vi "get User Info List.vi"(8 "error in (no error)":errorcluster, 11 "[Data] Abstruct Userinfo in":refnum<class "[Data] Abstruct Userinfo.lvclass">) -> (0 "error out":errorcluster, 2 "user info":T1(array[cluster]), 3 "[Data] Abstruct Userinfo out":refnum<class "[Data] Abstruct Userinfo.lvclass">)   [LabVIEW 2020, in "[Data] Abstruct Userinfo.lvclass"]
uses:
  [Data] Abstruct Userinfo.lvclass
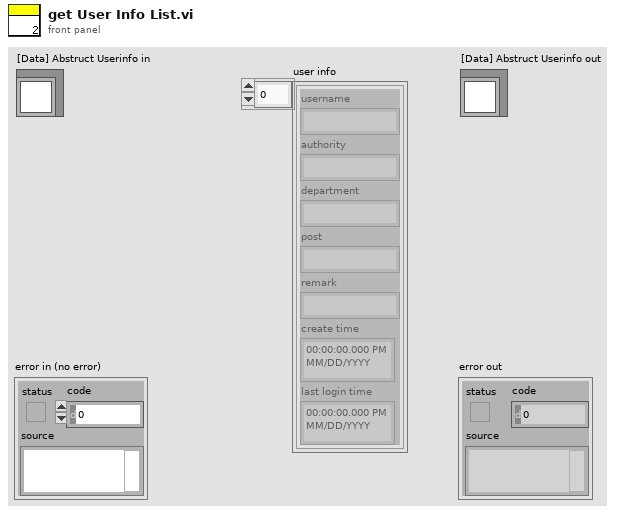
[diagram p1: front panel]
types:
  T1 = cluster{"username":string, "authority":string, "department":string, "post":string, "remark":string, "create time":timestamp, "last login time":timestamp}[]
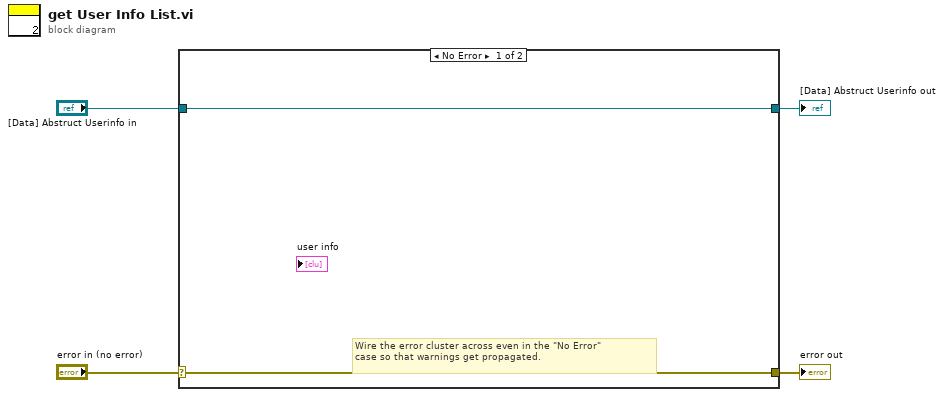
[diagram p0: block diagram]
diagram:
  n1 = case shown="No Error" "error in (no error)" {
    selector: "error in (no error)" -> [w5 w8]
    tunnel: [w5 w8] -> w3
    tunnel: [w6 w7] -> w1
    tunnel: "[Data] Abstruct Userinfo in" -> [w6 w7]
    frame No Error {
      # "Wire the error cluster across even in the \"No Error\"\ncase so that warnings get propagated."
    }
    frame Error {
    }
  }
  "error out" <- w3
  "[Data] Abstruct Userinfo out" <- w1
